vi "Write DebugTxt String.vi"(8 "error in (no error)":errorcluster, 11 "Input string":string) -> ()   [LabVIEW 2021, in "G5 Regatron Custom Device Engine.lvlib"]
uses:
  Engine/G5 Regatron Custom Device Engine.lvlib
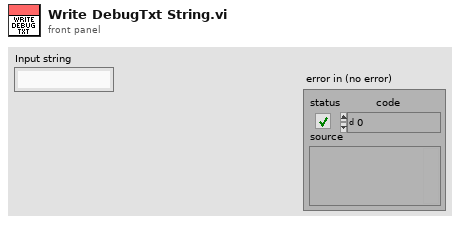
[diagram p1: front panel]
types:
  T1 = enum16{"open", "replace", "create", "open or create", "replace or create", "replace or create with confirmation"}
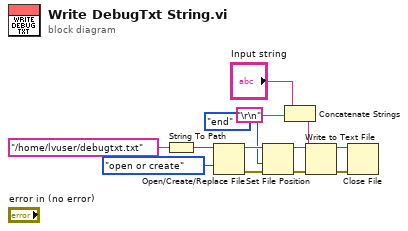
[diagram p0: block diagram]
diagram:
  n1 = String To Path(string="/home/lvuser/debugtxt.txt") -> (path=w8:path)
  n2 = Open/Create/Replace File(file path (use dialog)=w8, operation (0:open)=T1."open or create") -> (refnum out=w10:refnum<file>, error out=w12:errorcluster)  [unwired: 4 in, 1 out]
  n3 = Set File Position(refnum=w10, from (0:start)=enum16{"start", "end", "current"}."end", error in=w12) -> (refnum out=w11:refnum<file>, error out=w13:errorcluster)  [unwired: 1 in]
  n4 = Concatenate Strings("Input string", "\r\n") -> (w3:string)
  n5 = Write to Text File(file (use dialog)=w11, text=w3, error in=w13) -> (refnum out=w5:refnum<file>, error out=w4:errorcluster)  [unwired: 1 in, 1 out]
  n6 = Close File(refnum=w5, error in=w4) -> ()  [unwired: 2 out]
